vi "SwissSPAD Live_Bitfile Version.vi"(8 "error in (no error)":errorcluster, 11 "Bitfile Path":path) -> (0 "error out":errorcluster, 3 "Bitfile Version":string)   [LabVIEW 2021]
doc: "Reads a string from the bitfile header (Vivado version?)."
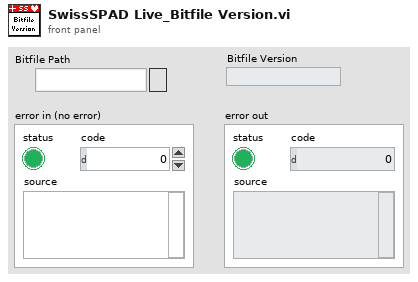
[diagram p1: front panel]
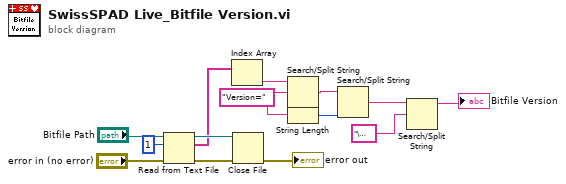
[diagram p0: block diagram]
diagram:
  w5 = "Version=" ("search string/char (-)")
  n1 = Read from Text File(file (use dialog)="Bitfile Path", count=1, error in="error in (no error)") -> (refnum out=w11:refnum<file>, text=w8:string[], error out=w10:errorcluster)  [unwired: 1 in, 1 out]
  n2 = Index Array(array=w8) -> (element=w7:string)  [unwired: 1 in]
  n3 = Close File(refnum=w11, error in=w10) -> (error out=→"error out":errorcluster)  [unwired: 1 out]
  n4 = Search/Split String(string=w7, search string/char (-)=w5) -> (match + rest of string=w6:string)  [unwired: 1 in, 2 out]
  n5 = String Length(string=w5) -> (length=w4:i32)
  n6 = Search/Split String(string=w6, offset (0)=w4) -> (match + rest of string=w3:string)  [unwired: 1 in, 2 out]
  n7 = Search/Split String(string=w3, search string/char (-)="\u0000" ("Bitfile Version")) -> (substring before match=→"Bitfile Version":string)  [unwired: 1 in, 2 out]
